vi "Instrument Level Processing.vi"(8 "error in (no error)":errorcluster, 9 "Instrument Level Controls in":variant, 10 "Voice Level Processing in":variant, 11 "MIDI Controls in":variant) -> (0 "error out":errorcluster, 2 "Instrument Level Processing out":variant)   [LabVIEW 2014, in "mySynthesizer.lvlib" / "Instrument Level Processing.lvlib"]
uses:
  Instrument Level Processing.lvlib
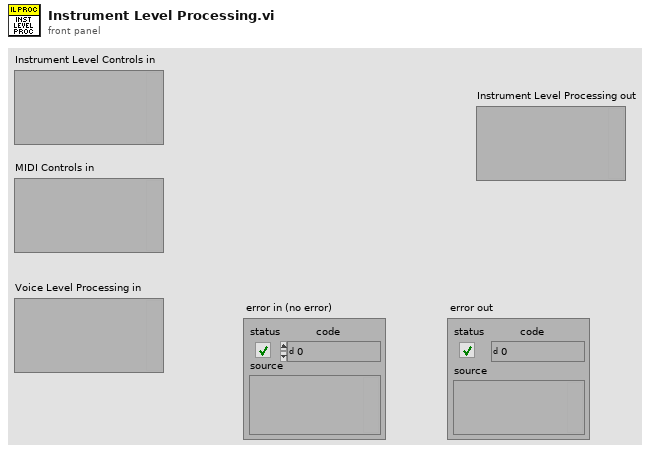
[diagram p1: front panel]
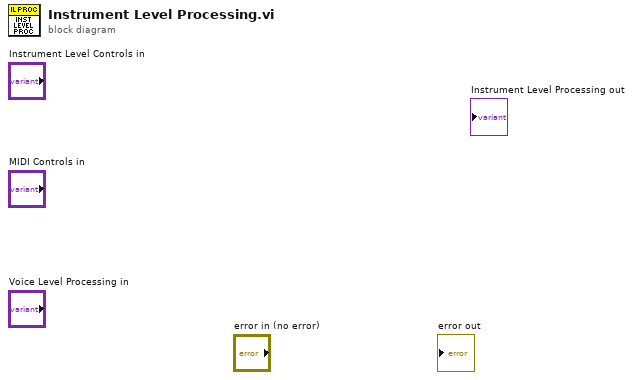
[diagram p0: block diagram]
diagram:
